vi "DriveAccel.vi"(0 "minMovePower":dbl, 1 "TargetPower":dbl, 2 "Ka":dbl, 5 "ForwardTicks":dbl, 7 "Direction":dbl, 9 "Kf":dbl, 11 "move":dbl, 12 "derivitive":dbl) -> (4 "pSpeed":dbl, 6 "Adjustment":dbl, 8 "RPower":dbl, 10 "LPower":dbl)   [LabVIEW 2017]
uses:
  Robot Global Data.vi
panel:
  out "previous_error":dbl
  out "error":dbl
  out "Kd":dbl
  out "WheelBreak":dbl
  out "xtime":dbl
  # "Inputs"
  # "Outputs"
  # "we need to add at the end: \nRPower = LPower = direction*WheelBrake;\n\tpSpeed = 0; \nsomehow"
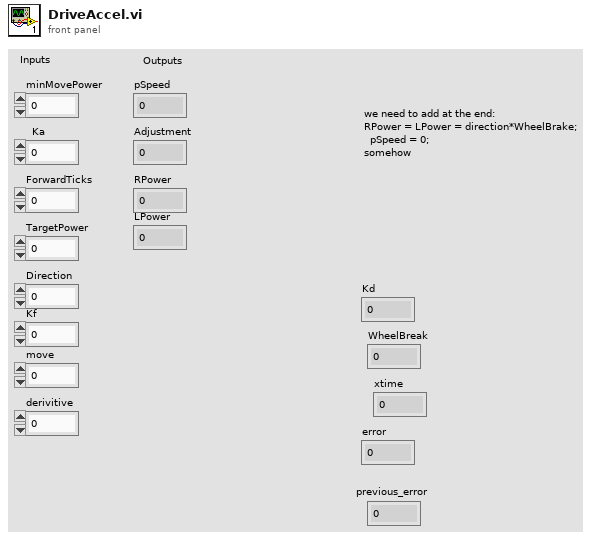
[diagram p1: front panel]
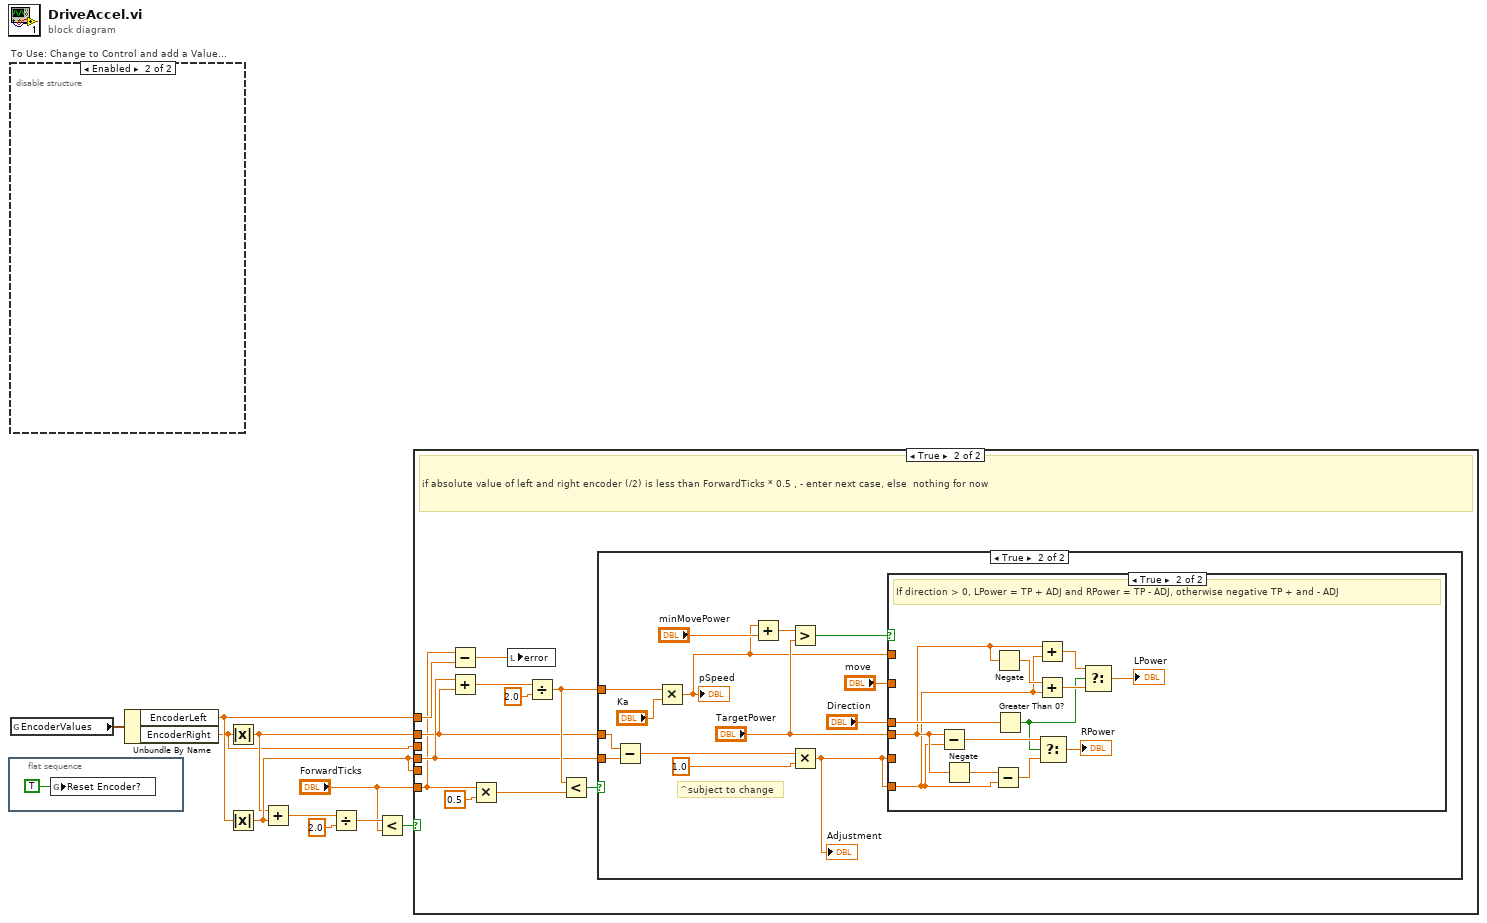
[diagram p0: block diagram]
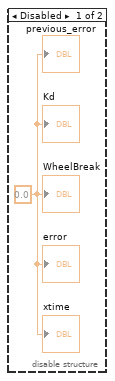
[diagram p2: hidden frame]
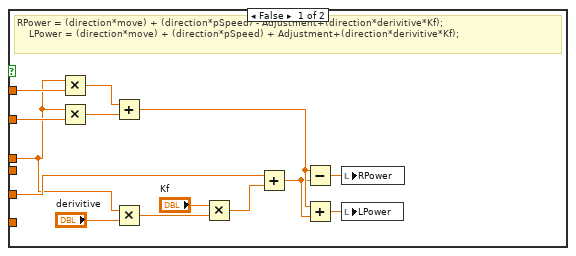
[diagram p5: hidden frame]
diagram:
  n1 = flat-sequence {
    frame #0 {
      n2 = global write "Robot Global Data.vi" "Reset Encoder?"(TRUE) -> ()
    }
  }
  n3 = disable-structure "To Use: Change to Control and add a Value..." shown="Enabled" {
    frame Disabled {
      w12 = 0.0
      "xtime" <- w12
      "previous_error" <- w12
      "error" <- w12
      "WheelBreak" <- w12
      "Kd" <- w12
    }
    frame Enabled {
    }
  }
  n4 = global read "Robot Global Data.vi" "EncoderValues"() -> (w6:cluster{"EncoderLeft":dbl, "EncoderRight":dbl})
  n5 = Unbundle By Name(w6) -> ("EncoderLeft"=w3:dbl, "EncoderRight"=w2:dbl)
  n6 = Absolute Value(x=w2) -> (abs(x)=w4:dbl)
  n7 = Absolute Value(x=w3) -> (abs(x)=w5:dbl)
  n8 = Add(x=w4, y=w5) -> (x+y=w9:dbl)
  n9 = Divide(x=w9, y=2.0) -> (x/y=w10:dbl)
  n10 = Less?(x=w10, y="ForwardTicks") -> (x < y?=w7:bool)
  n11 = case shown="True" w7 {
    tunnel: w3 -> [_ w22]
    tunnel: w5 -> [_ _]
    tunnel: w5 -> [_ w15]
    tunnel: w4 -> [_ w14]
    tunnel: w2 -> [_ _]
    tunnel: "ForwardTicks" -> [_ w13]
    frame False {
      # "BE DEPRESSED"
    }
    frame True {
      # "if absolute value of left and right encoder (/2) is less than ForwardTicks * 0.5 , - enter next case, else  nothing for now"
      n12 = Subtract(x=w13, y=w22) -> (x-y=w23:dbl)
      n13 = Add(x=w15, y=w14) -> (x+y=w21:dbl)
      n14 = Multiply(x=w13, y=0.5) -> (x*y=w18:dbl)
      n15 = local write "error"(w23) -> ()
      n16 = Divide(x=w21, y=2.0) -> (x/y=w16:dbl)
      n17 = Less?(x=w16, y=w18) -> (x < y?=w17:bool)
      n18 = case shown="True" w17 {
        tunnel: w16 -> [_ w37]
        tunnel: w14 -> [_ w34]
        tunnel: w15 -> [_ w35]
        frame False {
        }
        frame True {
          # "^subject to change"
          n19 = Subtract(x=w34, y=w35) -> (x-y=w33:dbl)
          n20 = Multiply(x=w37, y="Ka") -> (x*y=w25:dbl)
          "pSpeed" <- w25
          n21 = Add(x=w25, y="minMovePower") -> (x+y=w30:dbl)
          n22 = Greater?(x=w30, y="TargetPower") -> (0:w29:bool)
          n23 = Multiply(x=w33, y=1.0) -> (x*y=w24:dbl)
          "Adjustment" <- w24
          n24 = case shown="True" w29 {
            tunnel: "TargetPower" -> [_ w53]
            tunnel: w24 -> [_ w52]
            tunnel: "Direction" -> [w45 w63]
            tunnel: "move" -> [w51 _]
            tunnel: w25 -> [w49 _]
            tunnel: w24 -> [w47 _]
            frame False {
              # "RPower = (direction*move) + (direction*pSpeed) - Adjustment+(direction*derivitive*Kf);\n\t\t\t\tLPower = (direction*move) + (direction*pSpeed) + Adjustment+(direction*derivitive*Kf);"
              n25 = Multiply(x=w45, y=w49) -> (x*y=w48:dbl)
              n26 = Multiply(x=w45, y=w51) -> (x*y=w50:dbl)
              n27 = Add(x=w48, y=w50) -> (x+y=w41:dbl)
              n28 = Multiply(x=w45, y="derivitive") -> (x*y=w43:dbl)
              n29 = Multiply(x="Kf", y=w43) -> (x*y=w42:dbl)
              n30 = Add(x=w47, y=w42) -> (x+y=w40:dbl)
              n31 = Subtract(x=w41, y=w40) -> (x-y=w39:dbl)
              n32 = Add(x=w41, y=w40) -> (x+y=w38:dbl)
              n33 = local write "RPower"(w39) -> ()
              n34 = local write "LPower"(w38) -> ()
            }
            frame True {
              # "If direction > 0, LPower = TP + ADJ and RPower = TP - ADJ, otherwise negative TP + and - ADJ"
              n35 = Subtract(x=w53, y=w52) -> (x-y=w61:dbl)
              n36 = Negate(x=w53) -> (-x=w60:dbl)
              n37 = Subtract(x=w60, y=w52) -> (x-y=w59:dbl)
              n38 = Negate(x=w53) -> (-x=w57:dbl)
              n39 = Greater Than 0?(x=w63) -> (x > 0?=w54:bool)
              n40 = Add(x=w53, y=w52) -> (x+y=w56:dbl)
              n41 = Add(x=w57, y=w52) -> (x+y=w58:dbl)
              n42 = Select(t=w61, s=w54, f=w59) -> (s? t:f=→"RPower":dbl)
              n43 = Select(t=w56, s=w54, f=w58) -> (s? t:f=→"LPower":dbl)
            }
          }
        }
      }
    }
  }
